vi "host_logging_gm.vi"() -> ()   [LabVIEW 2011]
uses:
  <vilib>/addons/database/Connection.llb/Conn ObjectReference.ctl
  Output - Cluster gas.ctl
  gas_values.ctl
  <vilib>/Platform/TimedLoop/XDataNode/timing_clust.ctl
  <vilib>/Platform/TimedLoop/XDataNode/nitl_modes.ctl
  <vilib>/Platform/TimedLoop/XDataNode/wakeup.ctl
  <vilib>/Platform/TimedLoop/XDataNode/XDataNode.xnode
  <vilib>/Platform/TimedLoop/XDataNode/XDNodeRunTimeDep.lvlib
  <vilib>/addons/database/NI_Database_API.lvlib
panel:
  out "status":string
  in  "stop":bool caption="EXIT"
  out "Fehler":errorcluster
  in  "prefix for tables":string(combo)="GM"
  in  "interval [s]":u32=10 min=1 step=1
  in  "path":path
  # "GM DB Logging"
  # "database logging:"
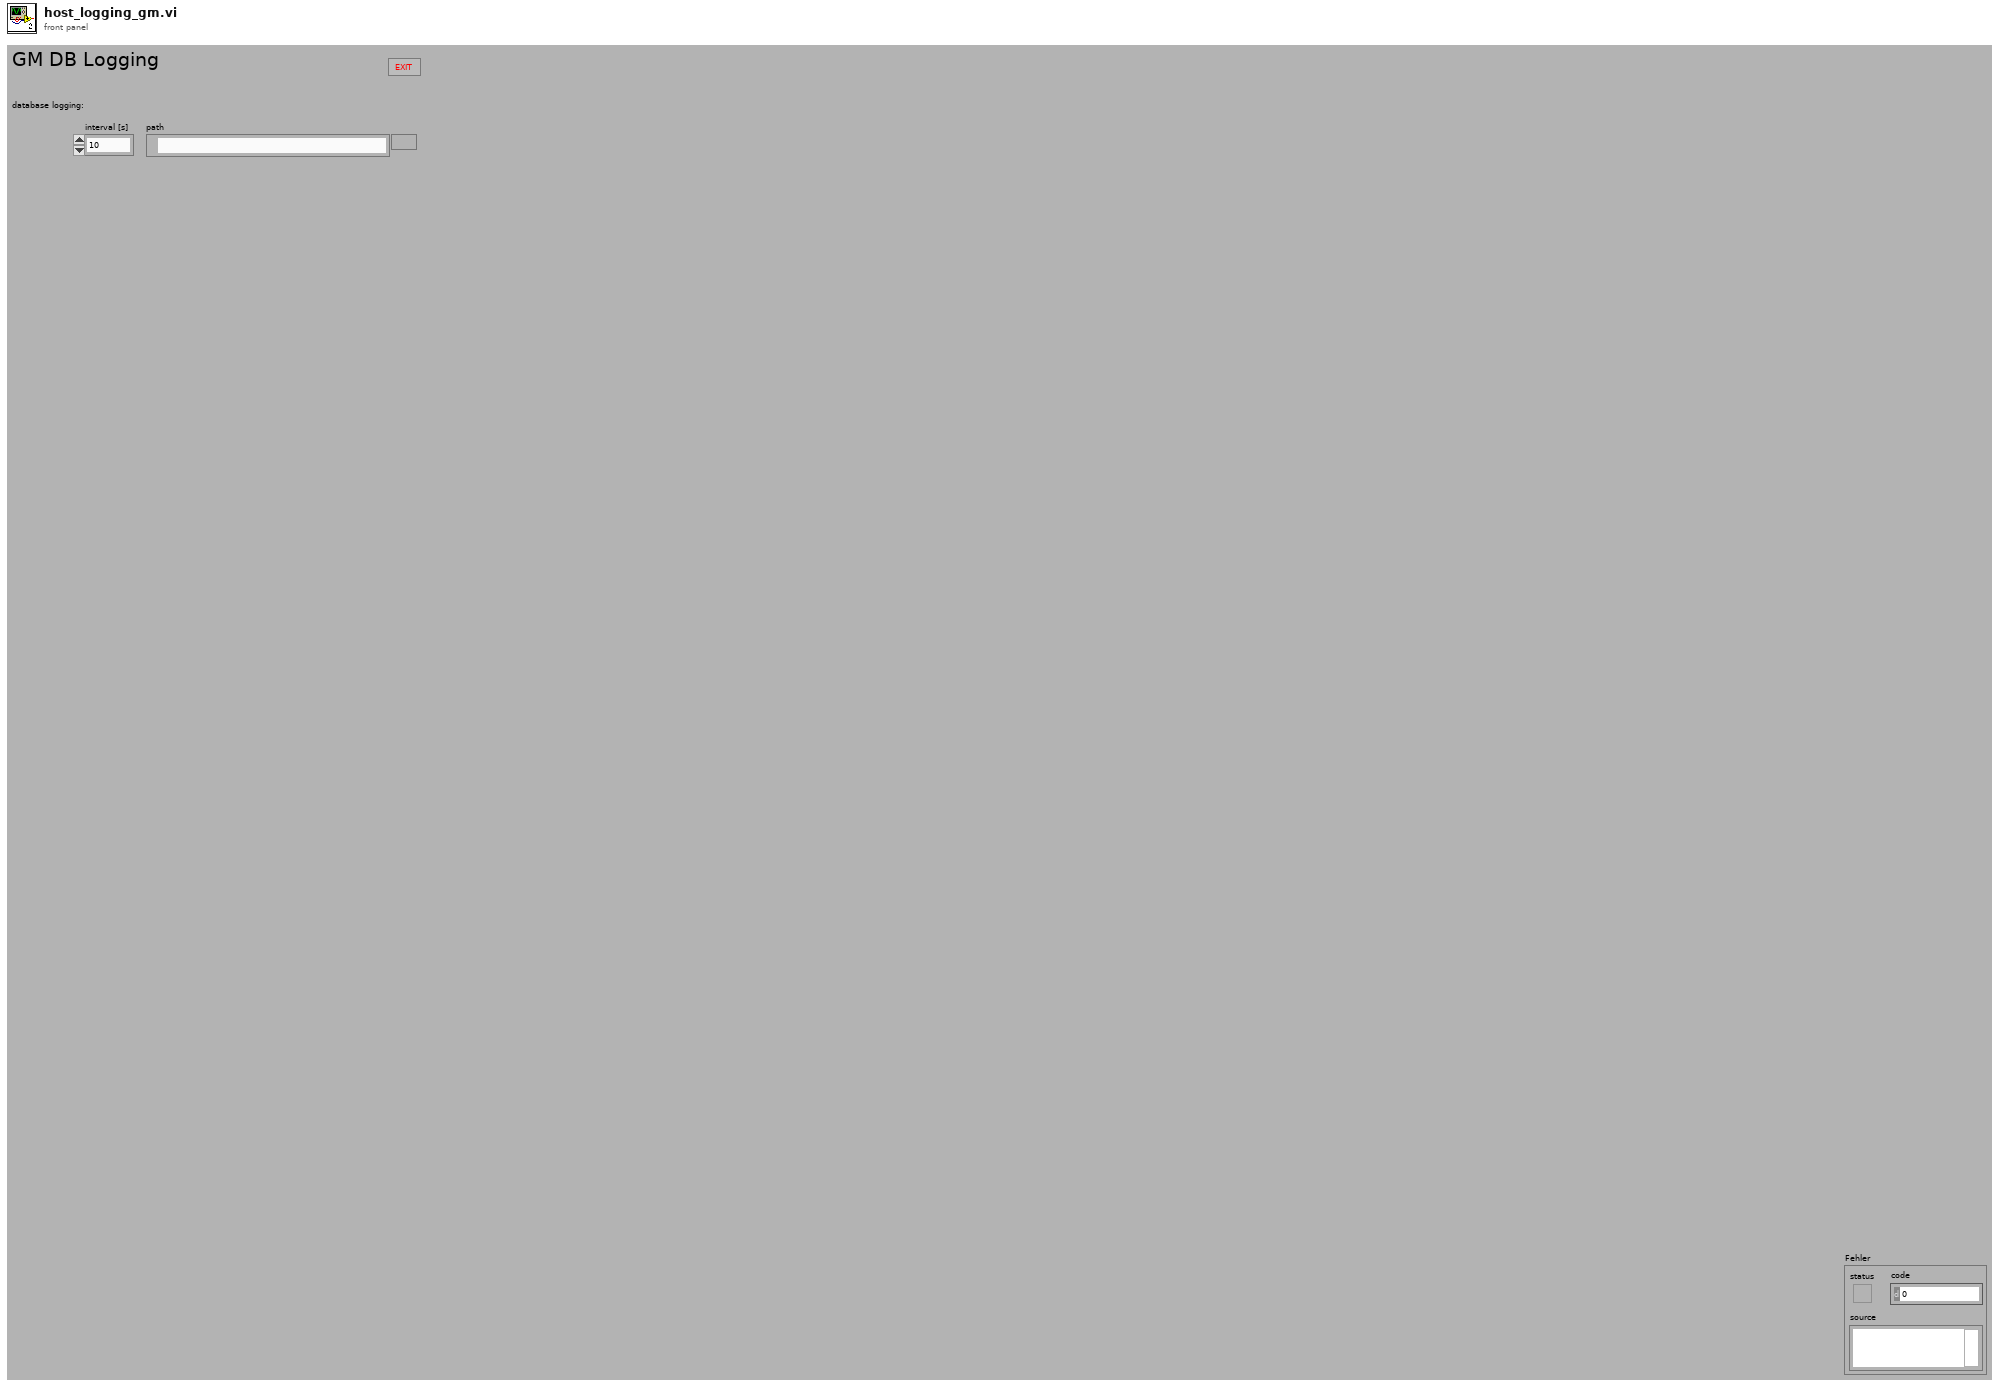
[diagram p1: front panel]
types:
  T1 = typedef "Output - Cluster gas.ctl" = cluster{"B2G2 MR V1.1 AUF":bool, "B2G2 MR V1.1 ZU":bool, "B2G2 MR V1 AUF":bool, "B2G2 MR V1 ZU":bool, "B2G1 T2 V1 AUF":bool, "B2G1 T2 V1 ZU":bool, "B2G1 T2 V1.1 AUF":bool, "B2G1 T2 V1.1 ZU":bool, "B2G2 T2 V1 AUF":bool, "B2G2 T2 V1 ZU":bool, "B2G2 T2 V1.1 ZU":bool, "B2G2 T2 V1.1 AUF":bool, "B2G1 MR V1 AUF":bool, "B2G1 MR V1 ZU":bool, "B2G1 MR V1.1 AUF":bool, "B2G1 MR V1.1 ZU":bool, "B2G1 HR V1 AUF":bool, "B2G1 HR V1 ZU":bool, "B2G1 HR V1.1 AUF":bool, "B2G1 HR V1.1 ZU":bool, "Fab1 HR V1 AUF":bool, "Fab1 HR V1 ZU":bool, "Fab1 HR V1.1 AUF":bool, "Fab1 HR V1.1 ZU":bool, "Fab1 MR V1 AUF":bool, "Fab1 MR V1 ZU":bool, "Fab1 MR V1.1 AUF":bool, "Fab1 MR V1.1 ZU":bool, "Fab1 BL V1 AUF":bool, "Fab1 BL V1 ZU":bool, "Fab1 BL V1.1 AUF":bool, "Fab1 BL V1.1 ZU":bool, "Fab2 HR V1 AUF":bool, "Fab2 HR V1 ZU":bool, "Fab2 HR V1.1 AUF":bool, "Fab2 HR V1.1 ZU":bool, "Fab2 MR V1 AUF":bool, "Fab2 MR V1 ZU":bool, "Fab2 MR V1.1 AUF":bool, "Fab2 MR V1.1 ZU":bool, "GA1 ch4 [%]":dbl, "GA1 co2 [%]":dbl, "GA1 h2 [%]":dbl, "GM P1 RUN":bool, "GM V-1 AUF":bool, "GM V-1 ZU":bool, "GM V-2 AUF":bool, "GM V-2 ZU":bool, "GM V-3 AUF":bool, "GM V-3 ZU":bool, "GM V-4 AUF":bool, "GM V-4 ZU":bool, "GM P2 RUN":bool, "GM GZ-1 [imp]":u32, "GM DS-2 [bar]":dbl, "GM DS-1 [bar]":dbl, "GM TS-1 [°C]":dbl, "GM TS-2[°C]":dbl, "gas_values":T2, "measuring mode":u8, "GM V-5":bool}
  T2 = typedef "gas_values.ctl" = cluster{"start":timestamp, "GM DS-2 [bar]":dbl, "GA1 ch4 [%]":dbl, "GA1 co2 [%]":dbl, "GA1 h2 [%]":dbl, "GM DS-1 [bar]":dbl, "GM TS-1 [°C]":dbl, "GM TS-2 [°C]":dbl, "GM GZ-1 [l]":dbl, "measuring point":u8, "end":timestamp, "empty":bool, "GM GZ-1 [l] 2":dbl, "GM TS-1 [°C] 2":dbl, "GM DS-1 [bar] 2":dbl, "GM DS-2 [bar] 2":dbl, "empty 2":bool, "measuring mode":u8}
  T3 = typedef "NI_Database_API.lvlib/Conn ObjectReference.ctl" = refnum<k1>
  T4 = cluster{"file timing":i64, "db timing":i64, "GZ1":u32, "db reference":T3, "P2 RUN":bool, "P1 RUN":bool, "db":bool, "data refnum":refnum<k21>, "measmode":u32, "prefix":string, "output cluster reading time":timestamp, "V1":bool, "V2":bool, "V3":bool, "V4":bool, "gas_values.timestamp":timestamp}
  T5 = typedef "XDNodeRunTimeDep.lvlib/timing_clust.ctl" = cluster{"Expected End [f-1]":u64, "Actual End [f-1]":u64, "Finished Late? [f-1]":bool, "Expected End [i-1]":u64, "Actual End [i-1]":u64, "Finished Late? [i-1]":bool, "Expected Start [i]":u64, "Actual Start [i]":u64, "Expected Start [f]":u64, "Actual Start [f]":u64, "Source Name":string, "Structure Name":string, "Period":i64, "Deadline":i64, "Offset":i64, "Start":i64, "Priority":i32, "Timeout":i32, "Mode":T6, "Wakeup Reason":T7, "Error":errorcluster, "Source Type":string, "Secondary Source Type":string, "Global End Time":u64, "Global Start Time":u64, "Frame Duration":u64, "Iteration Duration":u64, "Assigned CPU":i32, "I/O Scan Engine Mode":u32}
  T6 = typedef "XDNodeRunTimeDep.lvlib/nitl_modes.ctl" = enum32{"No Change", "Process missed periods, maintain original phase", "Discard missed periods, maintain original phase", "Process missed periods, ignore original phase", "Discard missed periods, ignore original phase"}
  T7 = typedef "XDNodeRunTimeDep.lvlib/wakeup.ctl" = enum32{"Normal", "Aborted", "Asynchronous wakeup", "Timing source error", "Timed loop error", "Timeout"}
  T8 = cluster{"start":timestamp, "end":timestamp, "measuring point":u8, "measuring mode":u8, "GA1 co2 [%]":dbl, "GA1 ch4 [%]":dbl, "GA1 h2 [%]":dbl, "GM GZ-1 [l]":dbl, "GM DS-1 [bar]":dbl, "GM TS-1 [°C]":dbl, "GM DS-2 [bar]":dbl, "empty":bool, "GM GZ-1 [l] 2":dbl, "GM DS-1 [bar] 2":dbl, "GM TS-1 [°C] 2":dbl, "GM DS-2 [bar] 2":dbl, "empty 2":bool, "GM TS-2 [°C]":dbl}
  T9 = enum32{"invalid app kind", "Development System", "Run Time System", "Student Edition", "Embedded LabVIEW", "Evaluation", "Custom"}
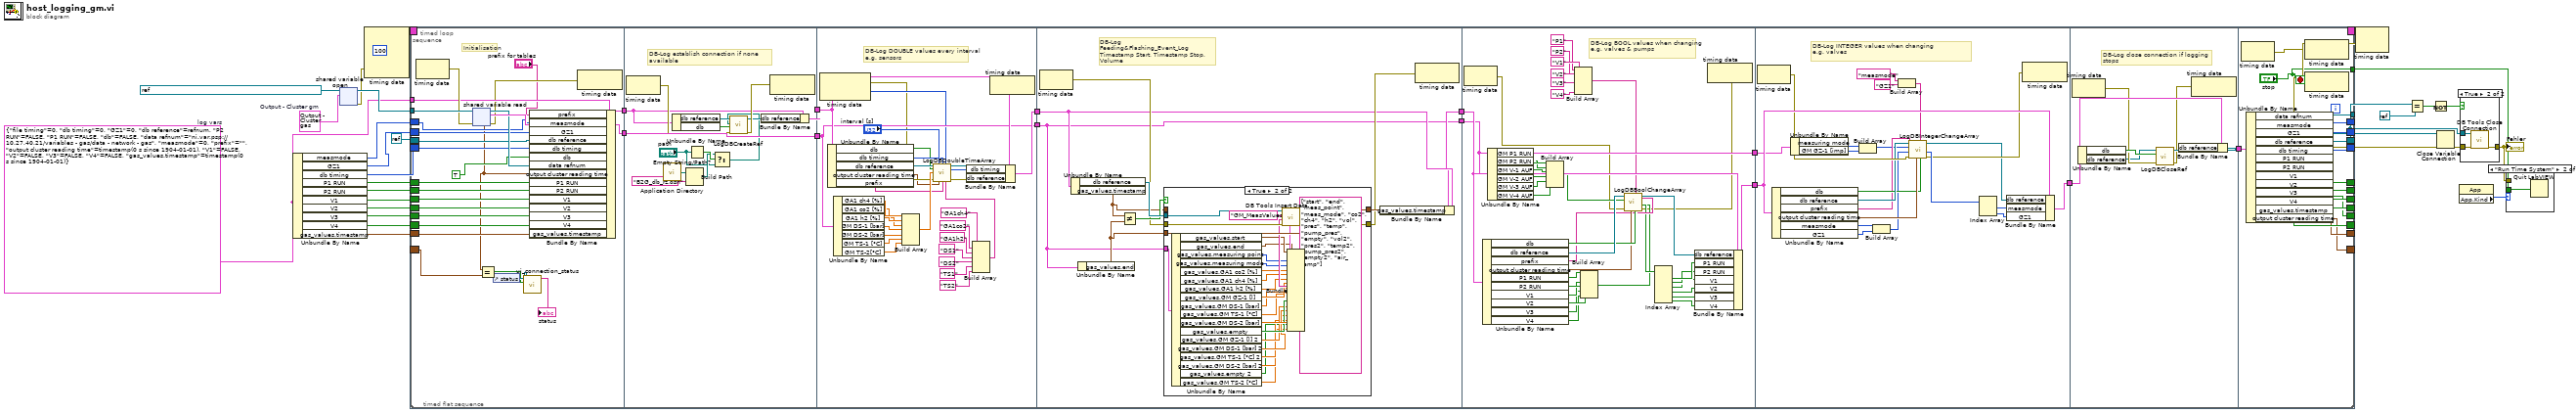
[diagram p0: block diagram]
diagram:
  w24 = T1 {"B2G2 MR V1.1 AUF"=FALSE, "B2G2 MR V1.1 ZU"=FALSE, "B2G2 MR V1 AUF"=FALSE, "B2G2 MR V1 ZU"=FALSE, "B2G1 T2 V1 AUF"=FALSE, "B2G1 T2 V1 ZU"=FALSE, "B2G1 T2 V1.1 AUF"=FALSE, "B2G1 T2 V1.1 ZU"=FALSE, "B2G2 T2 V1 AUF"=FALSE, "B2G2 T2 V1 ZU"=FALSE, "B2G2 T2 V1.1 ZU"=FALSE, "B2G2 T2 V1.1 AUF"=FALSE, "B2G1 MR V1 AUF"=FALSE, "B2G1 MR V1 ZU"=FALSE, "B2G1 MR V1.1 AUF"=FALSE, "B2G1 MR V1.1 ZU"=FALSE, "B2G1 HR V1 AUF"=FALSE, "B2G1 HR V1 ZU"=FALSE, "B2G1 HR V1.1 AUF"=FALSE, "B2G1 HR V1.1 ZU"=FALSE, "Fab1 HR V1 AUF"=FALSE, "Fab1 HR V1 ZU"=FALSE, "Fab1 HR V1.1 AUF"=FALSE, "Fab1 HR V1.1 ZU"=FALSE, "Fab1 MR V1 AUF"=FALSE, "Fab1 MR V1 ZU"=FALSE, "Fab1 MR V1.1 AUF"=FALSE, "Fab1 MR V1.1 ZU"=FALSE, "Fab1 BL V1 AUF"=FALSE, "Fab1 BL V1 ZU"=FALSE, "Fab1 BL V1.1 AUF"=FALSE, "Fab1 BL V1.1 ZU"=FALSE, "Fab2 HR V1 AUF"=FALSE, "Fab2 HR V1 ZU"=FALSE, "Fab2 HR V1.1 AUF"=FALSE, "Fab2 HR V1.1 ZU"=FALSE, "Fab2 MR V1 AUF"=FALSE, "Fab2 MR V1 ZU"=FALSE, "Fab2 MR V1.1 AUF"=FALSE, "Fab2 MR V1.1 ZU"=FALSE, "GA1 ch4 [%]"=0.0, "GA1 co2 [%]"=0.0, "GA1 h2 [%]"=0.0, "GM P1 RUN"=FALSE, "GM V-1 AUF"=FALSE, "GM V-1 ZU"=FALSE, "GM V-2 AUF"=FALSE, "GM V-2 ZU"=FALSE, "GM V-3 AUF"=FALSE, "GM V-3 ZU"=FALSE, "GM V-4 AUF"=FALSE, "GM V-4 ZU"=FALSE, "GM P2 RUN"=FALSE, "GM GZ-1 [imp]"=0, "GM DS-2 [bar]"=0.0, "GM DS-1 [bar]"=0.0, "GM TS-1 [°C]"=0.0, "GM TS-2[°C]"=0.0, "gas_values"={"start"=timestamp(0 s since 1904-01-01), "GM DS-2 [bar]"=0.0, "GA1 ch4 [%]"=0.0, "GA1 co2 [%]"=0.0, "GA1 h2 [%]"=0.0, "GM DS-1 [bar]"=0.0, "GM TS-1 [°C]"=0.0, "GM TS-2 [°C]"=0.0, "GM GZ-1 [l]"=0.0, "measuring point"=0, "end"=timestamp(0 s since 1904-01-01), "empty"=FALSE, "GM GZ-1 [l] 2"=0.0, "GM TS-1 [°C] 2"=0.0, "GM DS-1 [bar] 2"=0.0, "GM DS-2 [bar] 2"=0.0, "empty 2"=FALSE, "measuring mode"=0}, "measuring mode"=0, "GM V-5"=FALSE}  # Output - Cluster gm
  w12 = T4 {"file timing"=0, "db timing"=0, "GZ1"=0, "db reference"=refnum, "P2 RUN"=FALSE, "P1 RUN"=FALSE, "db"=FALSE, "data refnum"="ni.var.psp://10.27.40.21/variables - gas/data - network - gas", "measmode"=0, "prefix"="", "output cluster reading time"=timestamp(0 s since 1904-01-01), "V1"=FALSE, "V2"=FALSE, "V3"=FALSE, "V4"=FALSE, "gas_values.timestamp"=timestamp(0 s since 1904-01-01)}  # log vars
  n1 = Unbundle By Name(w12) -> ("measmode"=w7:u32, "GZ1"=w6:u32, "db timing"=w5:i64, "P1 RUN"=w11:bool, "P2 RUN"=w10:bool, "V1"=w9:bool, "V2"=w8:bool, "V3"=w4:bool, "V4"=w3:bool, "gas_values.timestamp"=w1:timestamp)
  n2 = shared-variable-open(refnum<k21> "ni.var.psp://10.27.40.21/variables - gm/data - network - gm" ("output variable"), w24) -> (w25:refnum<k21>, w22:errorcluster)  [unwired: 2 in]
  n3 = node-c288(i64 100 ("Period"), w22) -> (w29:T5)  [unwired: 2 in]
  n4 = timed-loop {
    timing: w29 -> [_]
    timing-out: [_] -> w28
    shift-right: [w56] -> _
    shift-left: w5 -> [w57]
    tunnel: w12 -> [w55]
    shift-right: [w47] -> _
    shift-left: w6 -> [w52]
    shift-right: [w46] -> w15
    shift-left: refnum<k0> refnum -> [w54]
    tunnel: w25 -> [w53]
    shift-right: [w51] -> _
    shift-left: w11 -> [w50]
    shift-right: [w49] -> _
    shift-left: w8 -> [w48]
    tunnel: [w45] -> w13
    shift-right: [w44] -> _
    shift-left: w10 -> [w43]
    shift-right: [w42] -> _
    shift-left: w9 -> [w41]
    shift-right: [w40] -> _
    shift-left: w7 -> [w39]
    shift-right: [w38] -> _
    shift-left: w3 -> [w37]
    shift-right: [w36] -> _
    shift-left: w4 -> [w35]
    tunnel: [w34] -> w2
    shift-right: [w33] -> _
    shift-left: w1 -> [w32]
    shift-right: [w31] -> _
    shift-left: _ -> [w30]
    stop <- "stop" stop-if-true
    n5 = timed-sequence {
      timing: _ -> [_]
      timing-out: _ -> [_]
      tunnel: w57 -> [w97]
      tunnel: [w96] -> w56
      tunnel: w55 -> [w95]
      tunnel: w54 -> [w94]
      tunnel: w53 -> [w89]
      tunnel: w52 -> [w88]
      tunnel: [w85] -> w51
      tunnel: w50 -> [w84]
      tunnel: [w83] -> w49
      tunnel: w48 -> [w82]
      tunnel: [w75] -> w47
      tunnel: [w74] -> w46
      tunnel: [w73] -> w45
      tunnel: [w72] -> w44
      tunnel: w43 -> [w71]
      tunnel: [w70] -> w42
      tunnel: w41 -> [w69]
      tunnel: [w68] -> w40
      tunnel: w39 -> [w67]
      tunnel: [w66] -> w38
      tunnel: w37 -> [w65]
      tunnel: [w64] -> w36
      tunnel: w35 -> [w63]
      tunnel: [w62] -> w34
      tunnel: [w61] -> w33
      tunnel: w32 -> [w60]
      tunnel: [w59] -> w31
      tunnel: w30 -> [w58]
      n6 = timed-flat-sequence {
        tunnel: w97 -> [w111]
        tunnel: [w120] -> w93
        tunnel: w95 -> [w114]
        tunnel: [w113] -> w91
        tunnel: w94 -> [w116]
        tunnel: w89 -> [w122]
        tunnel: w88 -> [w115]
        tunnel: w84 -> [w118]
        tunnel: w82 -> [w119]
        tunnel: w71 -> [w110]
        tunnel: w69 -> [w109]
        tunnel: w67 -> [w108]
        tunnel: w65 -> [w106]
        tunnel: w63 -> [w107]
        tunnel: w60 -> [w104]
        tunnel: w58 -> [w98]
        tunnel: w93 -> [w141]
        tunnel: [w141] -> w92
        tunnel: w91 -> [w137]
        tunnel: [w136] -> w90
        tunnel: w92 -> [w174]
        tunnel: [w174] -> w87
        tunnel: w90 -> [w175]
        tunnel: [w176] -> w86
        tunnel: w87 -> [w183]
        tunnel: [w183] -> w81
        tunnel: w86 -> [w184]
        tunnel: [w187] -> w80
        tunnel: w81 -> [w261]
        tunnel: w80 -> [w262]
        tunnel: [w263] -> w79
        tunnel: [w261] -> w76
        tunnel: w79 -> [w289]
        tunnel: [w290] -> w78
        tunnel: w76 -> [w271]
        tunnel: w78 -> [w301]
        tunnel: [w296] -> w77
        tunnel: [w317] -> w96
        tunnel: [w315] -> w85
        tunnel: [w312] -> w83
        tunnel: w77 -> [w322]
        tunnel: [w316] -> w75
        tunnel: [w318] -> w74
        tunnel: ["stop"] -> w73
        tunnel: [w314] -> w72
        tunnel: [w313] -> w70
        tunnel: [w319] -> w68
        tunnel: [w310] -> w66
        tunnel: [w311] -> w64
        tunnel: [w320] -> w62
        tunnel: [w309] -> w61
        tunnel: [w308] -> w59
        frame #0 {
          # "Initialisation"
          n7 = node-c288() -> (w121:errorcluster)  [unwired: 1 in]
          n8 = shared-variable-read(w122, w121) -> (w117:refnum<k21>, w112:errorcluster, w120:T1, w99:timestamp)
          n9 = Equal?(x=w99, y=w98) -> (x = y?=w100:bool)
          n10 = control-ref of="status"() -> (w101:refnum<vi>)
          n11 = call "ui_connection_status.vi"("Boolean"=w100, "String in"=w101) -> ("status"=→"status":string)  [unwired: 9 in]
          n12 = Bundle By Name(cluster=w114, "prefix"="prefix for tables", "measmode"=w108, "GZ1"=w115, "db reference"=w116, "db timing"=w111, "db"=TRUE ("on/off"), "data refnum"=w117, "output cluster reading time"=w99, "P1 RUN"=w118, "P2 RUN"=w110, "V1"=w109, "V2"=w119, "V3"=w107, "V4"=w106, "gas_values.timestamp"=w104) -> (w113:T4)
          n13 = node-c288(w112) -> ()  [unwired: 1 out]
        }
        frame #1 {
          # "DB-Log establish connection if none available"
          n14 = node-c288() -> (w139:errorcluster)  [unwired: 1 in]
          n15 = call <vilib>:"Application Directory.vi"() -> ("Application Directory"=w131:path)
          n16 = Unbundle By Name(w137) -> ("db reference"=w140:T3, "db"=w134:bool)
          n17 = Build Path(base path=w131, name or relative path="B2G_db_rz.dsn" ("Name of ini file 2")) -> (appended path=w132:path)
          n18 = Empty String/Path?(string/path="path") -> (empty?=w133:bool)
          n19 = Select(t=w132, s=w133, f="path") -> (s? t:f=w129:path)
          n20 = call "LogDBCreateRef.vi"("error in (no error)"=w139, "db"=w134, "Pfad in"=w129, "Refnum in"=w140) -> ("error out"=w138:errorcluster, "Refnum out"=w135:T3)  [unwired: 6 in]
          n21 = Bundle By Name(cluster=w137, "db reference"=w135) -> (w136:T4)
          n22 = node-c288(w138) -> ()  [unwired: 1 out]
        }
        frame #2 {
          # "DB-Log DOUBLE values every interval\ne.g. sensors"
          n23 = node-c288() -> (w155:errorcluster, w171:i64)  [unwired: 1 in]
          n24 = Unbundle By Name(w175) -> ("db"=w166:bool, "db timing"=w172:i64, "db reference"=w167:T3, "output cluster reading time"=w154:timestamp, "prefix"=w153:string)
          n25 = Unbundle By Name(w174) -> ("GA1 ch4 [%]"=w157:dbl, "GA1 co2 [%]"=w152:dbl, "GA1 h2 [%]"=w151:dbl, "GM DS-1 [bar]"=w150:dbl, "GM DS-2 [bar]"=w149:dbl, "GM TS-1 [°C]"=w148:dbl, "GM TS-2[°C]"=w147:dbl)
          n26 = Build Array(w157, w152, w151, w150, w149, w148, w147) -> (w156:dbl[])
          n27 = Build Array("GA1ch4" ("table"), "GA1co2" ("table"), "GA1h2" ("table"), "DS1" ("table"), "DS2" ("table"), "TS1" ("table"), "TS2" ("table")) -> (w158:string[])
          n28 = call "LogDBDoubleTimeArray.vi"("Refnum in"=w167, "db Interval [s]"="interval [s]", "db timing"=w172, "Actual Start [f] in"=w171, "db"=w166, "values"=w156, "error in (no error)"=w155, "Time Stamp"=w154, "prefix"=w153, "names"=w158) -> ("Refnum out"=w169:T3, "Actual Start [f] out"=w170:i64, "error out"=w168:errorcluster)  [unwired: 3 in]
          n29 = Bundle By Name(cluster=w175, "db timing"=w170, "db reference"=w169) -> (w176:T4)
          n30 = node-c288(w168) -> ()  [unwired: 1 out]
        }
        frame #3 {
          # "DB-Log\nFeeding&Flashing_Event_Log\nTimestamp Start, Timestamp Stop, Volume"
          n31 = node-c288() -> (w186:errorcluster)  [unwired: 1 in]
          n32 = Unbundle By Name(w184) -> ("db reference"=w192:T3, "gas_values.timestamp"=w189:timestamp)
          n33 = Unbundle By Name(w183) -> ("gas_values.end"=w188:timestamp)
          n34 = Not Equal?(x=w189, y=w188) -> (x != y?=w191:bool)
          n35 = case shown="True" w191 {
            tunnel: w186 -> [w193 w219]
            tunnel: [w193 w218] -> w185
            tunnel: w192 -> [_ w217]
            tunnel: [w194 w220] -> w190
            tunnel: w189 -> [w194 _]
            tunnel: w188 -> [_ w220]
            tunnel: w183 -> [_ w215]
            frame False {
            }
            frame True {
              n36 = Unbundle By Name(w215) -> ("gas_values.start"=w212:timestamp, "gas_values.end"=w211:timestamp, "gas_values.measuring point"=w210:u8, "gas_values.measuring mode"=w209:u8, "gas_values.GA1 co2 [%]"=w208:dbl, "gas_values.GA1 ch4 [%]"=w207:dbl, "gas_values.GA1 h2 [%]"=w206:dbl, "gas_values.GM GZ-1 [l]"=w205:dbl, "gas_values.GM DS-1 [bar]"=w204:dbl, "gas_values.GM TS-1 [°C]"=w203:dbl, "gas_values.GM DS-2 [bar]"=w202:dbl, "gas_values.empty"=w201:bool, "gas_values.GM GZ-1 [l] 2"=w200:dbl, "gas_values.GM DS-1 [bar] 2"=w199:dbl, "gas_values.GM TS-1 [°C] 2"=w198:dbl, "gas_values.GM DS-2 [bar] 2"=w197:dbl, "gas_values.empty 2"=w196:bool, "gas_values.GM TS-2 [°C]"=w195:dbl)
              n37 = Bundle("start"=w212, "end"=w211, "measuring point"=w210, "measuring mode"=w209, "GA1 co2 [%]"=w208, "GA1 ch4 [%]"=w207, "GA1 h2 [%]"=w206, "GM GZ-1 [l]"=w205, "GM DS-1 [bar]"=w204, "GM TS-1 [°C]"=w203, "GM DS-2 [bar]"=w202, "empty"=w201, "GM GZ-1 [l] 2"=w200, "GM DS-1 [bar] 2"=w199, "GM TS-1 [°C] 2"=w198, "GM DS-2 [bar] 2"=w197, "empty 2"=w196, "GM TS-2 [°C]"=w195) -> (w216:T8)  [unwired: 1 in]
              n38 = call <vilib>:"DB Tools Insert Data.vi"("data"=w216, "error in (no error)"=w219, "columns"=string[] ["start", "end", "meas_point", "meas_mode", "co2", "ch4", "h2", "vol", "pres", "temp", "pump_pres", "empty", "vol2", "pres2", "temp2", "pump_pres2", "empty2", "air_temp"], "table"="GM_MeasValues", "connection reference"=w217) -> ("error out"=w218:errorcluster)  [unwired: 5 in, 1 out]
            }
          }
          n39 = Bundle By Name(cluster=w184, "gas_values.timestamp"=w190) -> (w187:T4)
          n40 = node-c288(w185) -> ()  [unwired: 1 out]
        }
        frame #4 {
          # "DB-Log BOOL values when changing\ne.g. valves & pumps"
          n41 = node-c288() -> (w227:errorcluster)  [unwired: 1 in]
          n42 = Unbundle By Name(w262) -> ("db"=w252:bool, "db reference"=w253:T3, "prefix"=w250:string, "output cluster reading time"=w251:timestamp, "P1 RUN"=w241:bool, "P2 RUN"=w240:bool, "V1"=w239:bool, "V2"=w238:bool, "V3"=w237:bool, "V4"=w236:bool)
          n43 = Unbundle By Name(w261) -> ("GM P1 RUN"=w234:bool, "GM P2 RUN"=w233:bool, "GM V-1 AUF"=w232:bool, "GM V-2 AUF"=w231:bool, "GM V-3 AUF"=w230:bool, "GM V-4 AUF"=w229:bool)
          n44 = Build Array(w234, w233, w232, w231, w230, w229) -> (w228:bool[])
          n45 = Build Array("P1" ("table"), "P2" ("table"), "V1" ("table"), "V2" ("table"), "V3" ("table"), "V4" ("table")) -> (w254:string[])
          n46 = Build Array(w241, w240, w239, w238, w237, w236) -> (w235:bool[])
          n47 = call "LogDBBoolChangeArray.vi"("db"=w252, "names"=w254, "cluster reading time"=w251, "prefix"=w250, "error in (no error)"=w227, "shift reg in"=w235, "values"=w228, "db reference"=w253) -> ("error out"=w226:errorcluster, "shift reg out"=w248:bool[], "db reference out"=w249:T3)  [unwired: 1 in]
          n48 = Index Array(array=w248) -> (element #1=w247:bool, element #2=w246:bool, element #3=w245:bool, element #4=w244:bool, element #5=w243:bool, element #6=w242:bool)  [unwired: 6 in]
          n49 = Bundle By Name(cluster=w262, "db reference"=w249, "P1 RUN"=w247, "P2 RUN"=w246, "V1"=w245, "V2"=w244, "V3"=w243, "V4"=w242) -> (w263:T4)
          n50 = node-c288(w226) -> ()  [unwired: 1 out]
        }
        frame #5 {
          # "DB-Log INTEGER values when changing\ne.g. valves"
          n51 = node-c288() -> (w280:errorcluster)  [unwired: 1 in]
          n52 = Unbundle By Name(w289) -> ("db"=w275:bool, "db reference"=w277:T3, "prefix"=w270:string, "output cluster reading time"=w278:timestamp, "measmode"=w274:u32, "GZ1"=w273:u32)
          n53 = Unbundle By Name(w271) -> ("measuring mode"=w285:u8, "GM GZ-1 [imp]"=w284:u32)
          n54 = Build Array(w285, w284) -> (w269:u32[])
          n55 = Build Array(w274, w273) -> (w272:u32[])
          n56 = Build Array("measmode" ("table"), "GZ1" ("table")) -> (w286:string[])
          n57 = call "LogDBIntegerChangeArray.vi"("db"=w275, "names"=w286, "current time"=w278, "prefix"=w270, "error in (no error)"=w280, "shift reg in"=w272, "values"=w269, "Refnum in"=w277) -> ("error out"=w279:errorcluster, "shift reg out"=w281:u32[], "Refnum out"=w276:T3)  [unwired: 1 in]
          n58 = Index Array(array=w281) -> (element #1=w283:u32, element #2=w282:u32)  [unwired: 2 in]
          n59 = Bundle By Name(cluster=w289, "db reference"=w276, "measmode"=w283, "GZ1"=w282) -> (w290:T4)
          n60 = node-c288(w279) -> ()  [unwired: 1 out]
        }
        frame #6 {
          # "DB-Log close connection if logging stops"
          n61 = node-c288() -> (w299:errorcluster)  [unwired: 1 in]
          n62 = Unbundle By Name(w301) -> ("db"=w300:bool, "db reference"=w297:T3)
          n63 = call "LogDBCloseRef.vi"("error in (no error)"=w299, "enable"=w300, "Refnum in"=w297) -> ("error out"=w298:errorcluster, "Refnum out"=w302:T3)  [unwired: 7 in]
          n64 = Bundle By Name(cluster=w301, "db reference"=w302) -> (w296:T4)
          n65 = node-c288(w298) -> ()  [unwired: 1 out]
        }
        frame #7 {
          n66 = node-c288() -> (w323:errorcluster)  [unwired: 1 in]
          n67 = Unbundle By Name(w322) -> ("data refnum"=w320:refnum<k21>, "measmode"=w319:u32, "GZ1"=w316:u32, "db reference"=w318:T3, "db timing"=w317:i64, "P1 RUN"=w315:bool, "P2 RUN"=w314:bool, "V1"=w313:bool, "V2"=w312:bool, "V3"=w311:bool, "V4"=w310:bool, "gas_values.timestamp"=w309:timestamp, "output cluster reading time"=w308:timestamp)
          n68 = node-c288(w323) -> ()  [unwired: 1 out]
        }
      }
    }
    n69 = node-c288() -> ()  [unwired: 1 in, 1 out]
    n70 = node-c288() -> ()  [unwired: 1 in, 1 out]
  }
  n71 = node-c288(w28) -> (w14:errorcluster)
  n72 = Equal?(x=w15, y=refnum<k0> refnum) -> (x = y?=w21:bool)
  n73 = Not(x=w21) -> (.not. x?=w19:bool)
  n74 = Close Variable Connection(8:w14, 11:w2) -> (0:w18:errorcluster)
  n75 = property class="App"() -> ("App.Kind"=w17:T9)  [unwired: 2 in, 2 out]
  n76 = case shown="True" w19 {
    tunnel: w18 -> [w331 w334]
    tunnel: w15 -> [_ w333]
    tunnel: [w331 w332] -> w16
    frame False {
    }
    frame True {
      n77 = call <vilib>:"DB Tools Close Connection.vi"("error in (no error)"=w334, "connection reference"=w333) -> ("error out"=w332:errorcluster)  [unwired: 5 in]
    }
  }
  "Fehler" <- w16
  n78 = case shown="\"Run Time System\"" w17 {
    tunnel: w16 -> [_ _ _]
    tunnel: w13 -> [_ w335 _]
    frame "invalid app kind", Default {
    }
    frame "Run Time System" {
      n79 = Quit LabVIEW(quit? (T)=w335) -> ()
    }
    frame "Development System" {
    }
  }
